vi "ToolProgramTest.vi"(8 "error in (no error)":errorcluster, 11 "VISA resource name":refnum<visa-resource-name>="COM5") -> (0 "error out":errorcluster, 1 "read string 3":string, 2 "read string 2":string, 3 "read string":string, 4 "read string 6":string, 5 "Array":string[](array[string]))   [LabVIEW 2019]
panel:
  out "read string 13":string
  out "read string 12":string
  out "read string 11":string
  out "read string 10":string
  out "read string 9":string
  out "read string 8":string
  out "read string 5":string
  out "read string 4":string
  in  "stop":bool
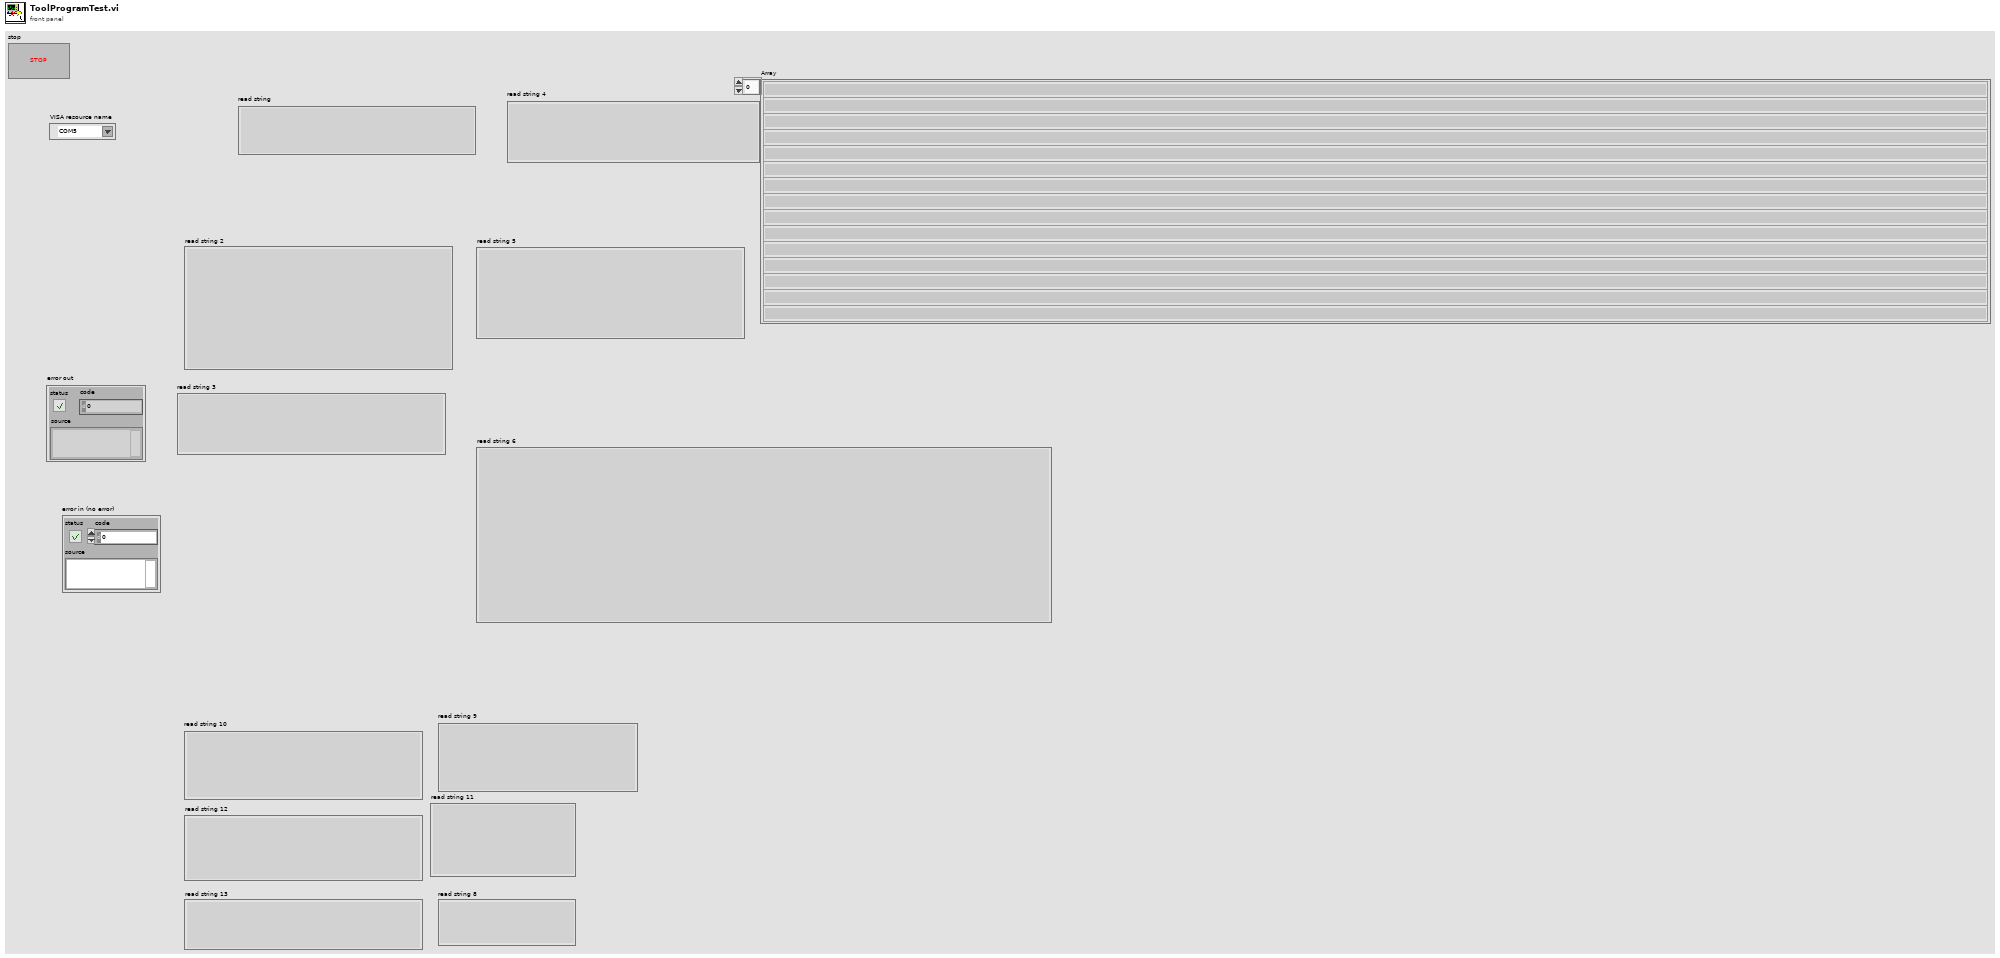
[diagram p1: front panel]
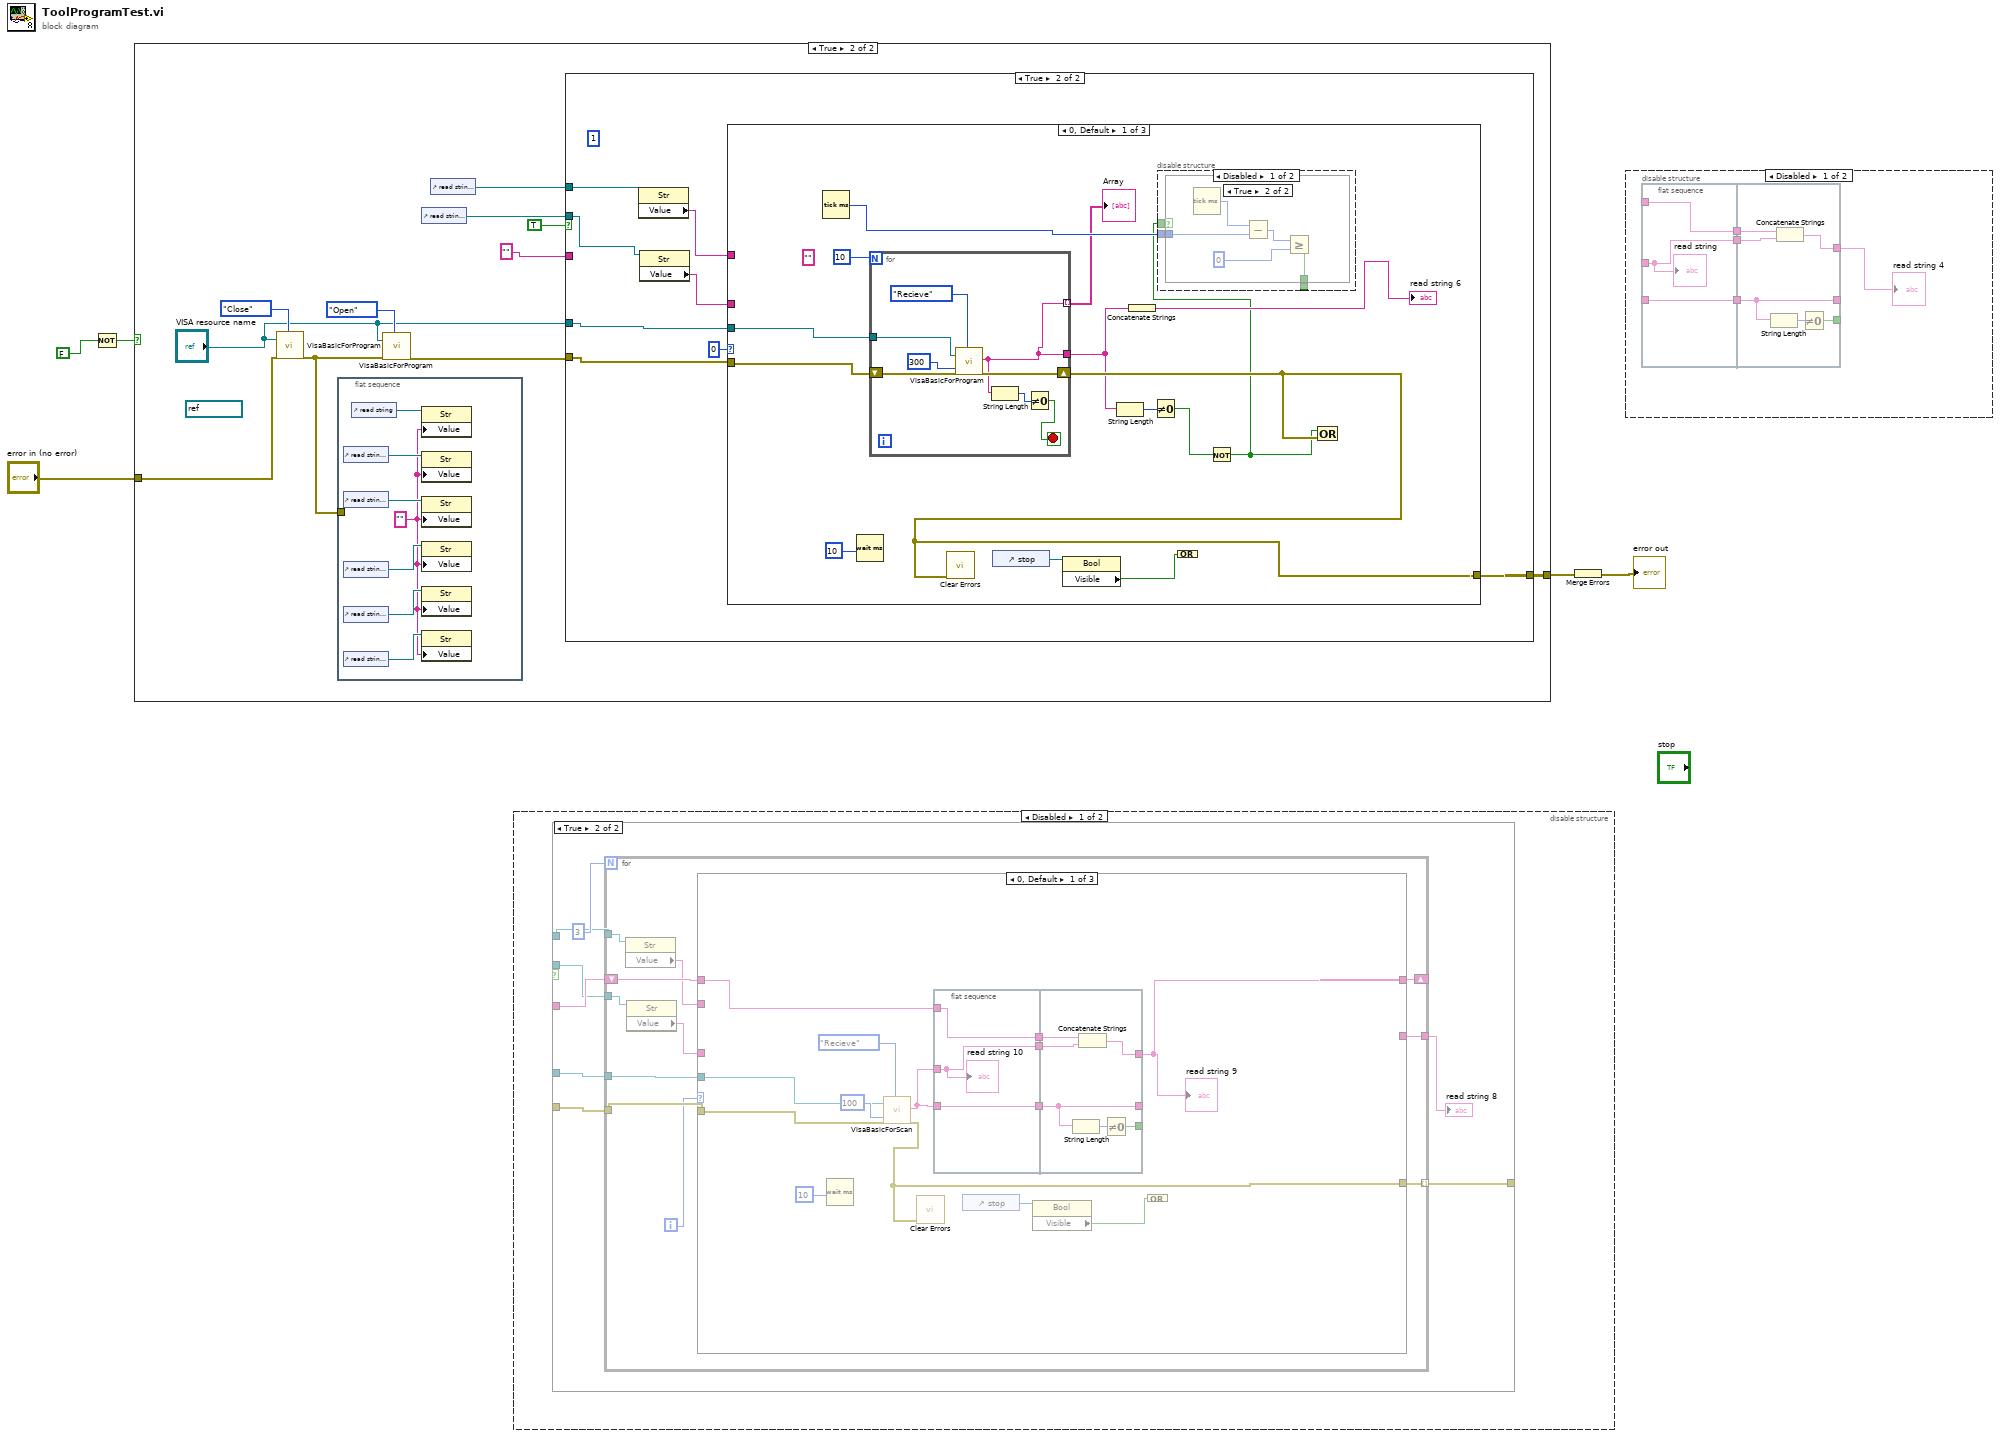
[diagram p0: block diagram]
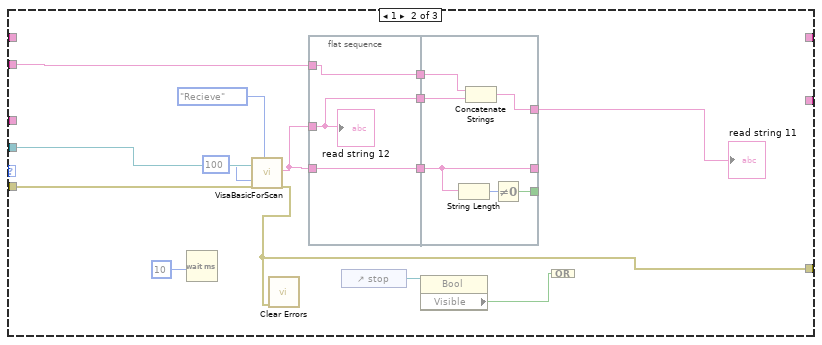
[diagram p4: hidden frame]
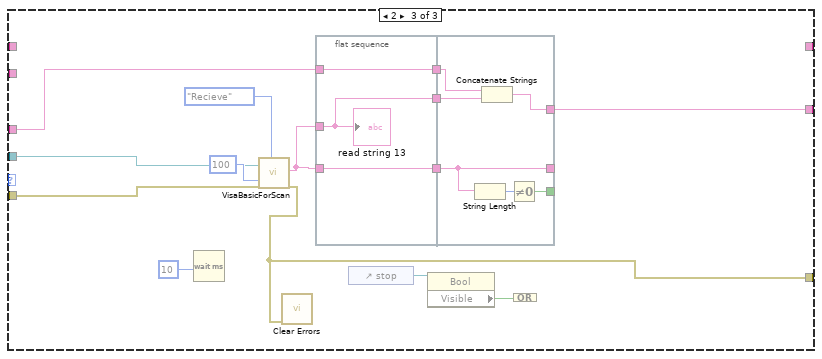
[diagram p5: hidden frame]
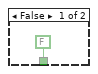
[diagram p9: hidden frame]
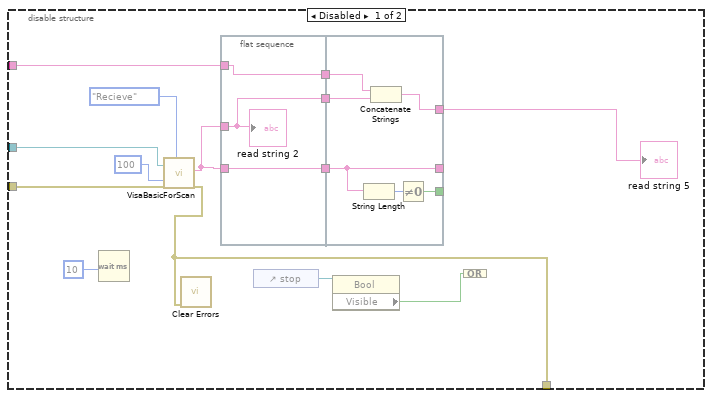
[diagram p12: hidden frame]
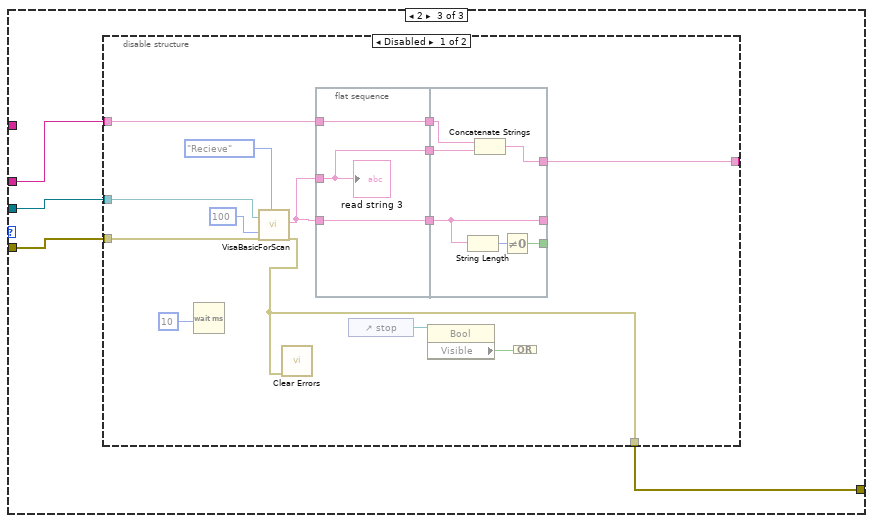
[diagram p13: hidden frame]
diagram:
  n1 = Not(x=FALSE) -> (.not. x?=w4:bool)
  n2 = case shown="True" w4 {
    tunnel: [_ w7] -> w3
    tunnel: "error in (no error)" -> [_ w6]
    frame False {
    }
    frame True {
      (unwired) refnum<visa-resource-name> "COM5" ("VISA resource name")
      n3 = call "VisaBasicForProgram.vi"("VISA resource name"="VISA resource name", "error in (no error)"=w6, "VisaAction"=enum16{"Open", "Send", "Recieve", "Close"}."Close") -> ("error out"=w12:errorcluster)  [unwired: 15 in, 1 out]
      n4 = flat-sequence {
        tunnel: w12 -> [_]
        frame #0 {
          w17 = "" ("read string")
          n5 = control-ref of="read string 2"() -> (w21:refnum<vi>)
          n6 = control-ref of="read string 3"() -> (w22:refnum<vi>)
          n7 = control-ref of="read string 4"() -> (w20:refnum<vi>)
          n8 = control-ref of="read string 5"() -> (w19:refnum<vi>)
          n9 = control-ref of="read string 6"() -> (w18:refnum<vi>)
          n10 = control-ref of="read string"() -> (w23:refnum<vi>)
          n11 = property class="Str"(reference=w23, "Value"=w17) -> ()  [unwired: 1 in, 2 out]
          n12 = property class="Str"(reference=w21, "Value"=w17) -> ()  [unwired: 1 in, 2 out]
          n13 = property class="Str"(reference=w22, "Value"=w17) -> ()  [unwired: 1 in, 2 out]
          n14 = property class="Str"(reference=w20, "Value"=w17) -> ()  [unwired: 1 in, 2 out]
          n15 = property class="Str"(reference=w19, "Value"=w17) -> ()  [unwired: 1 in, 2 out]
          n16 = property class="Str"(reference=w18, "Value"=w17) -> ()  [unwired: 1 in, 2 out]
        }
      }
      n17 = call "VisaBasicForProgram.vi"("VISA resource name"="VISA resource name", "error in (no error)"=w12, "VisaAction"=enum16{"Open", "Send", "Recieve", "Close"}."Open") -> ("error out"=w14:errorcluster)  [unwired: 15 in, 1 out]
      n18 = control-ref of="read string 5"() -> (w10:refnum<vi>)
      n19 = control-ref of="read string 4"() -> (w11:refnum<vi>)
      n20 = case shown="True" TRUE {
        tunnel: w14 -> [_ w31]
        tunnel: "VISA resource name" -> [_ w30]
        tunnel: "" ("read string") -> [_ _]
        tunnel: w11 -> [_ w29]
        tunnel: w10 -> [_ w28]
        tunnel: [_ w27] -> w7
        frame False {
        }
        frame True {
          (unwired) 1
          n21 = property class="Str"(reference=w29) -> ("Value"=w26:string)  [unwired: 1 in, 2 out]
          n22 = property class="Str"(reference=w28) -> ("Value"=w25:string)  [unwired: 1 in, 2 out]
          n23 = case shown="0, Default" 0 {
            tunnel: w31 -> [w41 w66 w93]
            tunnel: w30 -> [w42 w65 w94]
            tunnel: w26 -> [_ w64 _]
            tunnel: w25 -> [_ _ w92]
            tunnel: [w40 w63 w91] -> w27
            frame 0, Default {
              (unwired) "" ("read string")
              n24 = Tick Count (ms)() -> (millisecond timer value=w39:u32)
              n25 = Wait (ms)(milliseconds to wait=10) -> ()  [unwired: 1 out]
              n26 = for {
                N: 10 -> [_]
                tunnel: w42 -> [w53]
                tunnel: [w48] -> w35
                shift-right: [w51] -> w40
                shift-left: w41 -> [w52]
                tunnel: [w48] -> w32 mode=indexing
                stop <- w46 stop-if-true
                n27 = call "VisaBasicForProgram.vi"("VISA resource name"=w53, "Time(0.1)"=u32 300, "error in (no error)"=w52, "VisaAction"=enum16{"Open", "Send", "Recieve", "Close"}."Recieve") -> ("read string"=w48:string, "error out"=w51:errorcluster)  [unwired: 14 in]
                n28 = String Length(string=w48) -> (length=w47:i32)
                n29 = Not Equal To 0?(x=w47) -> (x != 0?=w46:bool)
              }
              "Array" <- w32
              n30 = call <vilib>:"Clear Errors.vi"("error in (no error)"=w40) -> ()  [unwired: 5 in, 2 out]
              n31 = control-ref of="stop"() -> (w45:refnum<vi>)
              n32 = property class="Bool"(reference=w45) -> ("Visible"=w44:bool)  [unwired: 1 in, 2 out]
              n33 = String Length(string=w35) -> (length=w37:i32)
              n34 = Concatenate Strings(w35) -> (→"read string 6":string)
              n35 = Not Equal To 0?(x=w37) -> (x != 0?=w36:bool)
              n36 = Compound Arithmetic op=OR(w44) -> ()  [unwired: 1 out]
              n37 = Not(x=w36) -> (.not. x?=w34:bool)
              n38 = disable-structure shown="Disabled" {
                disable-tunnel: w39 -> [w56 _]
                disable-tunnel: w34 -> [w55 _]
                disable-tunnel: [w54 _] -> _
                frame Disabled {
                  n39 = case shown="True" w55 {
                    tunnel: w56 -> [_ w61]
                    tunnel: [FALSE w58] -> w54
                    frame False {
                    }
                    frame True {
                      n40 = Tick Count (ms)() -> (millisecond timer value=w62:u32)
                      n41 = Subtract(x=w62, y=w61) -> (x-y=w60:u32)
                      n42 = Greater Or Equal?(x=w60, y=0) -> (x >= y?=w58:bool)
                    }
                  }
                }
                frame Enabled {
                }
              }
              n43 = Compound Arithmetic op=OR(w34, w40) -> ()  [unwired: 1 out]
            }
            frame 1 {
              n44 = disable-structure shown="Enabled" {
                disable-tunnel: w66 -> [w77 _]
                disable-tunnel: w65 -> [w76 _]
                disable-tunnel: w64 -> [w69 w90]
                disable-tunnel: [w67 _] -> w63
                disable-tunnel: [_ w90] -> _
                frame Disabled {
                  n45 = Wait (ms)(milliseconds to wait=10) -> ()  [unwired: 1 out]
                  n46 = call "VisaBasicForScan.vi"("VISA resource name"=w76, "Time(0.1)"=u32 100, "error in (no error)"=w77, "VisaAction"=enum16{"Open", "Send", "Recieve", "Close"}."Recieve") -> ("read string"=w73:string, "error out"=w67:errorcluster)  [unwired: 14 in]
                  n47 = call <vilib>:"Clear Errors.vi"("error in (no error)"=w67) -> ()  [unwired: 5 in, 2 out]
                  n48 = flat-sequence {
                    tunnel: w73 -> [w82]
                    tunnel: w73 -> [w83]
                    tunnel: [w83] -> w80
                    tunnel: [w81] -> w79
                    tunnel: [w82] -> w78
                    tunnel: w69 -> [w81]
                    tunnel: w80 -> [w87]
                    tunnel: [w87] -> _
                    tunnel: [w88] -> _
                    tunnel: [w86] -> w68
                    tunnel: w79 -> [w85]
                    tunnel: w78 -> [w84]
                    frame #0 {
                      "read string 2" <- w82
                    }
                    frame #1 {
                      n49 = String Length(string=w87) -> (length=w89:i32)
                      n50 = Concatenate Strings(w85, w84) -> (w86:string)
                      n51 = Not Equal To 0?(x=w89) -> (x != 0?=w88:bool)
                    }
                  }
                  n52 = control-ref of="stop"() -> (w72:refnum<vi>)
                  n53 = property class="Bool"(reference=w72) -> ("Visible"=w71:bool)  [unwired: 1 in, 2 out]
                  n54 = Compound Arithmetic op=OR(w71) -> ()  [unwired: 1 out]
                  "read string 5" <- w68
                }
                frame Enabled {
                }
              }
            }
            frame 2 {
              n55 = disable-structure shown="Disabled" {
                disable-tunnel: w94 -> [w99 _]
                disable-tunnel: w93 -> [w98 _]
                disable-tunnel: w92 -> [w97 _]
                disable-tunnel: [w96 _] -> _
                disable-tunnel: [w95 _] -> w91
                frame Disabled {
                  n56 = Wait (ms)(milliseconds to wait=10) -> ()  [unwired: 1 out]
                  n57 = call "VisaBasicForScan.vi"("VISA resource name"=w99, "Time(0.1)"=u32 100, "error in (no error)"=w98, "VisaAction"=enum16{"Open", "Send", "Recieve", "Close"}."Recieve") -> ("read string"=w105:string, "error out"=w95:errorcluster)  [unwired: 14 in]
                  n58 = call <vilib>:"Clear Errors.vi"("error in (no error)"=w95) -> ()  [unwired: 5 in, 2 out]
                  n59 = flat-sequence {
                    tunnel: w105 -> [w110]
                    tunnel: w105 -> [w111]
                    tunnel: [w111] -> w108
                    tunnel: [w110] -> w107
                    tunnel: w97 -> [w109]
                    tunnel: [w109] -> w106
                    tunnel: w108 -> [w115]
                    tunnel: [w115] -> _
                    tunnel: [w116] -> _
                    tunnel: [w114] -> w96
                    tunnel: w107 -> [w113]
                    tunnel: w106 -> [w112]
                    frame #0 {
                      "read string 3" <- w110
                    }
                    frame #1 {
                      n60 = String Length(string=w115) -> (length=w117:i32)
                      n61 = Concatenate Strings(w112, w113) -> (w114:string)
                      n62 = Not Equal To 0?(x=w117) -> (x != 0?=w116:bool)
                    }
                  }
                  n63 = control-ref of="stop"() -> (w104:refnum<vi>)
                  n64 = property class="Bool"(reference=w104) -> ("Visible"=w103:bool)  [unwired: 1 in, 2 out]
                  n65 = Compound Arithmetic op=OR(w103) -> ()  [unwired: 1 out]
                }
                frame Enabled {
                }
              }
            }
          }
        }
      }
    }
  }
  n66 = disable-structure shown="Disabled" {
    frame Disabled {
      n67 = case shown="True" {
        selector: _ -> [_ _]
        tunnel: _ -> [_ w125]
        tunnel: _ -> [_ w124]
        tunnel: _ -> [_ w123]
        tunnel: _ -> [_ w121]
        tunnel: _ -> [_ w120]
        tunnel: [_ w118] -> _
        frame False {
        }
        frame True {
          n68 = for {
            N: 3 -> [_]
            tunnel: w125 -> [w136]
            tunnel: w124 -> [w135]
            shift-right: [w132] -> _
            shift-left: w123 -> [w133]
            tunnel: w121 -> [w131]
            tunnel: w120 -> [w130]
            tunnel: [w127] -> w119
            tunnel: [w126] -> w118 mode=indexing
            i -> [w134]
            n69 = property class="Str"(reference=w131) -> ("Value"=w129:string)  [unwired: 1 in, 2 out]
            n70 = property class="Str"(reference=w130) -> ("Value"=w128:string)  [unwired: 1 in, 2 out]
            n71 = case shown="0, Default" w134 {
              tunnel: w136 -> [w142 w173 w188]
              tunnel: w135 -> [w143 w172 w189]
              tunnel: w129 -> [_ w162 _]
              tunnel: w128 -> [_ _ w186]
              tunnel: w133 -> [w139 _ _]
              tunnel: [w138 _ _] -> w132
              tunnel: [_ _ w184] -> w127
              tunnel: [w137 w160 w183] -> w126
              frame 0, Default {
                n72 = Wait (ms)(milliseconds to wait=10) -> ()  [unwired: 1 out]
                n73 = call "VisaBasicForScan.vi"("VISA resource name"=w143, "Time(0.1)"=u32 100, "error in (no error)"=w142, "VisaAction"=enum16{"Open", "Send", "Recieve", "Close"}."Recieve") -> ("read string"=w147:string, "error out"=w137:errorcluster)  [unwired: 14 in]
                n74 = call <vilib>:"Clear Errors.vi"("error in (no error)"=w137) -> ()  [unwired: 5 in, 2 out]
                n75 = flat-sequence {
                  tunnel: w147 -> [w151]
                  tunnel: w147 -> [w153]
                  tunnel: [w153] -> w150
                  tunnel: w139 -> [w152]
                  tunnel: [w152] -> w141
                  tunnel: [w151] -> w140
                  tunnel: w150 -> [w157]
                  tunnel: [w157] -> _
                  tunnel: [w158] -> _
                  tunnel: [w156] -> w138
                  tunnel: w141 -> [w155]
                  tunnel: w140 -> [w154]
                  frame #0 {
                    "read string 10" <- w151
                  }
                  frame #1 {
                    n76 = String Length(string=w157) -> (length=w159:i32)
                    n77 = Concatenate Strings(w155, w154) -> (w156:string)
                    n78 = Not Equal To 0?(x=w159) -> (x != 0?=w158:bool)
                  }
                }
                n79 = control-ref of="stop"() -> (w146:refnum<vi>)
                n80 = property class="Bool"(reference=w146) -> ("Visible"=w145:bool)  [unwired: 1 in, 2 out]
                n81 = Compound Arithmetic op=OR(w145) -> ()  [unwired: 1 out]
                "read string 9" <- w138
              }
              frame 1 {
                n82 = Wait (ms)(milliseconds to wait=10) -> ()  [unwired: 1 out]
                n83 = call "VisaBasicForScan.vi"("VISA resource name"=w172, "Time(0.1)"=u32 100, "error in (no error)"=w173, "VisaAction"=enum16{"Open", "Send", "Recieve", "Close"}."Recieve") -> ("read string"=w168:string, "error out"=w160:errorcluster)  [unwired: 14 in]
                n84 = call <vilib>:"Clear Errors.vi"("error in (no error)"=w160) -> ()  [unwired: 5 in, 2 out]
                n85 = flat-sequence {
                  tunnel: w168 -> [w175]
                  tunnel: w168 -> [w176]
                  tunnel: [w176] -> w171
                  tunnel: [w174] -> w164
                  tunnel: [w175] -> w163
                  tunnel: w162 -> [w174]
                  tunnel: w171 -> [w180]
                  tunnel: [w180] -> _
                  tunnel: [w181] -> _
                  tunnel: [w179] -> w161
                  tunnel: w164 -> [w178]
                  tunnel: w163 -> [w177]
                  frame #0 {
                    "read string 12" <- w175
                  }
                  frame #1 {
                    n86 = String Length(string=w180) -> (length=w182:i32)
                    n87 = Concatenate Strings(w178, w177) -> (w179:string)
                    n88 = Not Equal To 0?(x=w182) -> (x != 0?=w181:bool)
                  }
                }
                n89 = control-ref of="stop"() -> (w167:refnum<vi>)
                n90 = property class="Bool"(reference=w167) -> ("Visible"=w166:bool)  [unwired: 1 in, 2 out]
                n91 = Compound Arithmetic op=OR(w166) -> ()  [unwired: 1 out]
                "read string 11" <- w161
              }
              frame 2 {
                n92 = Wait (ms)(milliseconds to wait=10) -> ()  [unwired: 1 out]
                n93 = call "VisaBasicForScan.vi"("VISA resource name"=w189, "Time(0.1)"=u32 100, "error in (no error)"=w188, "VisaAction"=enum16{"Open", "Send", "Recieve", "Close"}."Recieve") -> ("read string"=w195:string, "error out"=w183:errorcluster)  [unwired: 14 in]
                n94 = call <vilib>:"Clear Errors.vi"("error in (no error)"=w183) -> ()  [unwired: 5 in, 2 out]
                n95 = flat-sequence {
                  tunnel: w195 -> [w198]
                  tunnel: w195 -> [w199]
                  tunnel: [w199] -> w196
                  tunnel: [w198] -> w187
                  tunnel: w186 -> [w197]
                  tunnel: [w197] -> w185
                  tunnel: w196 -> [w203]
                  tunnel: [w203] -> _
                  tunnel: [w204] -> _
                  tunnel: [w202] -> w184
                  tunnel: w187 -> [w201]
                  tunnel: w185 -> [w200]
                  frame #0 {
                    "read string 13" <- w198
                  }
                  frame #1 {
                    n96 = String Length(string=w203) -> (length=w205:i32)
                    n97 = Concatenate Strings(w200, w201) -> (w202:string)
                    n98 = Not Equal To 0?(x=w205) -> (x != 0?=w204:bool)
                  }
                }
                n99 = control-ref of="stop"() -> (w194:refnum<vi>)
                n100 = property class="Bool"(reference=w194) -> ("Visible"=w193:bool)  [unwired: 1 in, 2 out]
                n101 = Compound Arithmetic op=OR(w193) -> ()  [unwired: 1 out]
              }
            }
          }
          "read string 8" <- w119
        }
      }
    }
    frame Enabled {
    }
  }
  n102 = Merge Errors(w3) -> (→"error out":errorcluster)
  n103 = disable-structure shown="Disabled" {
    frame Disabled {
      n104 = flat-sequence {
        tunnel: _ -> [w210]
        tunnel: _ -> [w212]
        tunnel: [w212] -> w209
        tunnel: _ -> [w211]
        tunnel: [w211] -> w208
        tunnel: [w210] -> w207
        tunnel: w209 -> [w216]
        tunnel: [w216] -> _
        tunnel: [w217] -> _
        tunnel: [w215] -> w206
        tunnel: w208 -> [w214]
        tunnel: w207 -> [w213]
        frame #0 {
          "read string" <- w210
        }
        frame #1 {
          n105 = String Length(string=w216) -> (length=w218:i32)
          n106 = Concatenate Strings(w214, w213) -> (w215:string)
          n107 = Not Equal To 0?(x=w218) -> (x != 0?=w217:bool)
        }
      }
      "read string 4" <- w206
    }
    frame Enabled {
    }
  }
